vi "ODE-Circuit.vi"() -> ()   [LabVIEW 2023]
doc: "This example demonstrates how to use the polymorphic ODE solver in both Formula String mode and VI mode. Note that VI mode allows for setting constant values via front panel controls, and the formula is passed by reference from a separate VI (CircuitRHS.vi). CircuitRHS.vi contains the formula in LabVIEW code of the Circuit ODE system model:\n\ndi2/dt = (-(R1+R2)i2 - R1i3 + Vin)/L1\n\ndi3/dt = (-R1i2 - R1i3 + Vin)/L2\n\nSee the circuit diagram on the front panel of this VI."
uses:
  <vilib>/Simulation/Utility/Implementation/Shared/SIM Diagram Parameters.ctl
  <vilib>/Simulation/Implementation/Shared/SIM Continuous Solvers.ctl
  <vilib>/gmath/ode.llb/ODE Solver formula string.vi
  <vilib>/gmath/ode.llb/ODE Solver main.vi
  <vilib>/gmath/NI_Gmath.lvlib
panel:
  out "Current vs. Time":cluster{"times":dbl[], dbl[]}[](graph)
  in  "Stop":bool
  in  "Constants":T1={"R1"=1.0, "R2"=1.0, "L1"=1.0, "L2"=2.0, "Vin"=12.0}
  in  "Initial Conditions for variables (i2, i3)":dbl[](array[numeric])=[0.0, 0.0]
  in  "Formula String Parameters":T2={"ODE Right Hand Side"=["(Vin-(R1+R2)*i2-R1*i3)/L1", "(Vin-R1*i2-R1*i3)/L2"], "X (name of variables)"=["i2", "i3"], "time"="t"}
  # "Overview: This example demonstrates how to use the polymorphic ODE solver in both Formula String mode and VI mode for the Circuit Model below.\nRequirements: LabVIEW Full Development System\nInstructions: \n1. Run the VI.\n2. Modify the input parameters for the ODE solver(s).\n3. Click Stop to stop the VI."
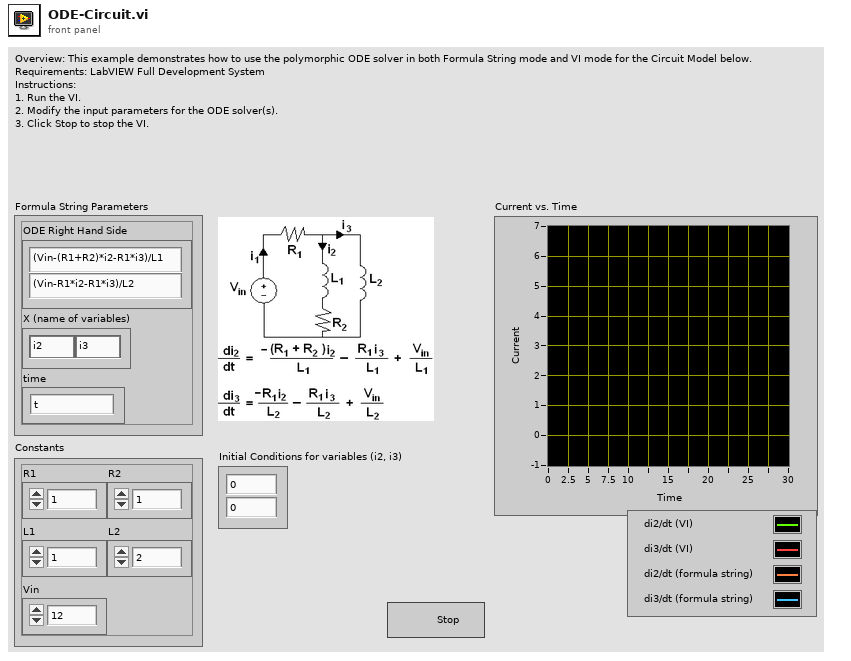
[diagram p1: front panel]
types:
  T1 = cluster{"R1":dbl, "R2":dbl, "L1":dbl, "L2":dbl, "Vin":dbl}
  T2 = cluster{"ODE Right Hand Side":string[], "X (name of variables)":string[], "time":string}
  T3 = typedef "SIM Diagram Parameters.ctl" = cluster{"Initial Time":dbl, "Final Time":dbl, "Time Step":dbl, "Absolute Tolerance":dbl, "Relative Tolerance":dbl, "Continuous Solver":T4, "Discrete Time Step":dbl, "Minimum Time Step":dbl, "Maximum Time Step":dbl, "Initial Time Step":dbl}
  T4 = typedef "SIM Continuous Solvers.ctl" = enum16{"Runge-Kutta 1 (Euler)", "Runge-Kutta 2", "Runge-Kutta 3", "Runge-Kutta 4", "Runge-Kutta 23 (variable)", "Runge-Kutta 45 (variable)", "BDF (variable)", "Adams-Moulton (variable)", "Rosenbrock (variable)", "Discrete States Only"}
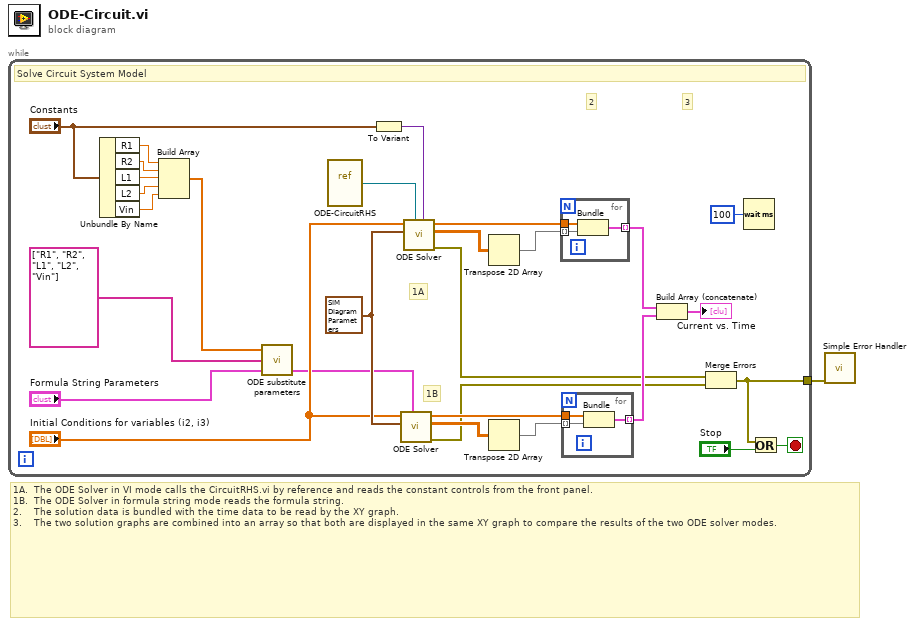
[diagram p0: block diagram]
diagram:
  # "1A.  The ODE Solver in VI mode calls the CircuitRHS.vi by reference and reads the constant controls from the front panel.\n1B.  The ODE Solver in formula string mode reads the formula string.\n2.    The solution data is bundled with the time data to be read by the XY graph.\n3.    The two solution graphs are combined into an array so that both are displayed in the same XY graph to compare the results of the two ODE solver modes."
  n1 = while {
    tunnel: [w4] -> w1
    stop <- w5 stop-if-true
    w26 = T3 {"Initial Time"=0.0, "Final Time"=30.0, "Time Step"=0.1, "Absolute Tolerance"=0.001, "Relative Tolerance"=1e-06, "Continuous Solver"=enum."Adams-Moulton (variable)", "Discrete Time Step"=2.0, "Minimum Time Step"=1e-06, "Maximum Time Step"=1.0, "Initial Time Step"=0.01} ("Simulation Parameters")
    # "3"
    # "1B"
    # "2"
    # "1A"
    # "Solve Circuit System Model"
    n2 = Unbundle By Name("Constants") -> ("R1"=w12:dbl, "R2"=w11:dbl, "L1"=w10:dbl, "L2"=w9:dbl, "Vin"=w8:dbl)
    n3 = Build Array(w12, w11, w10, w9, w8) -> (w7:dbl[])
    n4 = call "ODE substitute parameters.vi"("Formula String Parameters"="Formula String Parameters", "parameters"=string[] ["R1", "R2", "L1", "L2", "Vin"], "values"=w7) -> ("Formula String Parameters with substitutions"=w14:T2)  [unwired: 2 out]
    n5 = vi-ref "ODE-CircuitRHS.vi"() -> ("vi reference"=w30:refnum<vi>)
    n6 = To Variant(anything="Constants") -> (Variant=w18:variant)
    n7 = call-poly <vilib>:"ODE Solver.vi"("ODE RHS"=w14, "simulation parameters"=w26, "x0"="Initial Conditions for variables (i2, i3)") -> ("error out"=w3:errorcluster, "outputs"=w21:dbl[][], "times"=w25:dbl[])  [unwired: 1 in, 5 out]
    n8 = call-poly <vilib>:"ODE Solver.vi"("data"=w18, "ODE F(X,t)"=w30, "simulation parameters"=w26, "x0"="Initial Conditions for variables (i2, i3)") -> ("error out"=w2:errorcluster, "outputs"=w27:dbl[][], "times"=w28:dbl[])  [unwired: 1 in, 4 out]
    n9 = Transpose 2D Array(2D array=w27) -> (transposed array=w29:dbl[][])
    n10 = Transpose 2D Array(2D array=w21) -> (transposed array=w22:dbl[][])
    n11 = for {
      tunnel: w29 -> [w36] mode=indexing
      tunnel: w28 -> [w35]
      tunnel: [w34] -> w20 mode=indexing
      n12 = Bundle("times"=w35, w36) -> (w34:cluster{"times":dbl[], dbl[]})  [unwired: 1 out]
    }
    n13 = for {
      tunnel: w22 -> [w33] mode=indexing
      tunnel: w25 -> [w32]
      tunnel: [w31] -> w24 mode=indexing
      n14 = Bundle("times"=w32, w33) -> (w31:cluster{"times":dbl[], dbl[]})  [unwired: 1 out]
    }
    n15 = Build Array (concatenate)(w20, w24) -> (→"Current vs. Time":cluster{"times":dbl[], dbl[]}[])
    n16 = Merge Errors(w2, w3) -> (w4:errorcluster)
    n17 = Wait (ms)(milliseconds to wait=u32 100 ("millisecond multiple")) -> ()  [unwired: 1 out]
    n18 = Or(x=w4, y="Stop") -> (x .or. y?=w5:bool)
  }
  n19 = call <vilib>:"Simple Error Handler.vi"("error in (no error)"=w1) -> ()  [unwired: 4 in, 5 out]
